vi "Compute Strike Velocity.vi"(3 "drag coefficient":sgl format="%.5f", 4 "decay distance":sgl format="%.3f", 5 "raw velocity":sgl format="%.3f", 6 "distance units":string="FOOT") -> (0 "conversion factor":sgl format="%.5f", 1 "correction factor":sgl=1.0 format="%.4f", 2 "strike velocity":sgl format="%.3f")   [LabVIEW 2015]
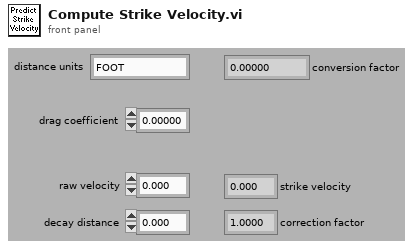
[diagram p1: front panel]
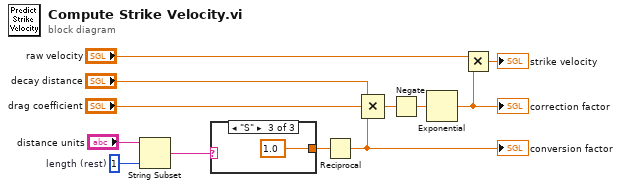
[diagram p0: block diagram]
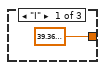
[diagram p2: hidden frame]
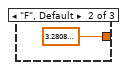
[diagram p3: hidden frame]
diagram:
  w11 = 1  # length (rest)
  n1 = String Subset(string="distance units", length (rest)=w11) -> (substring=w10:string)  [unwired: 1 out]
  n2 = case shown="\"S\"" w10 {
    tunnel: [sgl 39.37 sgl 3.2808 sgl 1.0] -> w6
    frame "I" {
    }
    frame "F", Default {
    }
    frame "S" {
    }
  }
  n3 = Reciprocal(x=w6) -> (1/x=w3:sgl)
  "conversion factor" <- w3
  n4 = Compound Arithmetic op=MULTIPLY("decay distance", "drag coefficient", w3) -> (w9:sgl)
  n5 = Negate(x=w9) -> (-x=w8:sgl)
  n6 = Exponential(1:w8) -> (0:w1:sgl)
  "correction factor" <- w1
  n7 = Multiply(x="raw velocity", y=w1) -> (x*y=→"strike velocity":sgl)
